vi "Exclude Servo Errors.vi"(10 "Group Names":string[](array[string])) -> (2 "Group Names Out":string[](array[string]))   [LabVIEW 2013]
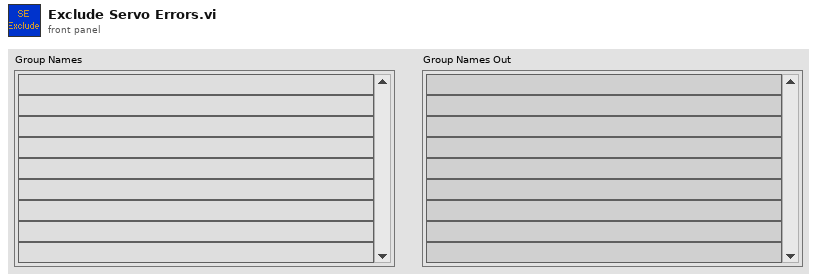
[diagram p1: front panel]
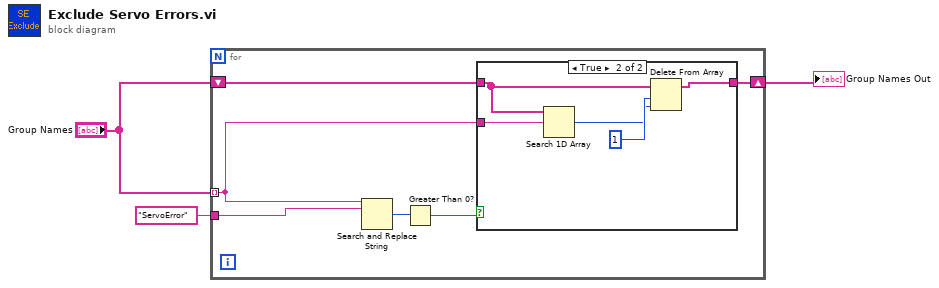
[diagram p0: block diagram]
diagram:
  n1 = for {
    tunnel: "Group Names" -> [w6] mode=indexing
    tunnel: "ServoError" ("String") -> [w7]
    shift-right: [w4] -> w1
    shift-left: "Group Names" -> [w5]
    n2 = Search and Replace String(input string=w6, search string=w7) -> (number of replacements=w9:i32)  [unwired: 6 in, 3 out]
    n3 = Greater Than 0?(x=w9) -> (x > 0?=w8:bool)
    n4 = case shown="True" w8 {
      tunnel: w6 -> [_ w12]
      tunnel: w5 -> [w10 w13]
      tunnel: [w10 w14] -> w4
      frame False {
      }
      frame True {
        n5 = Search 1D Array(1D array=w13, element=w12) -> (index of element=w11:i32)  [unwired: 1 in]
        n6 = Delete From Array(array=w13, length=1, index=w11) -> (array with subset deleted=w14:string[])  [unwired: 1 out]
      }
    }
  }
  "Group Names Out" <- w1
